vi "SerialPortTest.vi"() -> ()   [LabVIEW 2013]
panel:
  out "error out 2":errorcluster
  out "Buffer":string
  out "error out":errorcluster
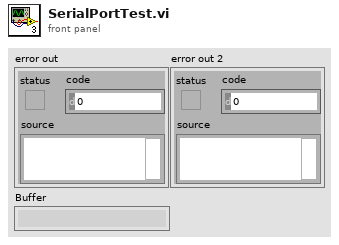
[diagram p1: front panel]
types:
  T1 = typedef "WPI_SerialPortRef.ctl" = cluster{"DevStatus":errorcluster, "Serial Port Name":refnum<visa-resource-name>}
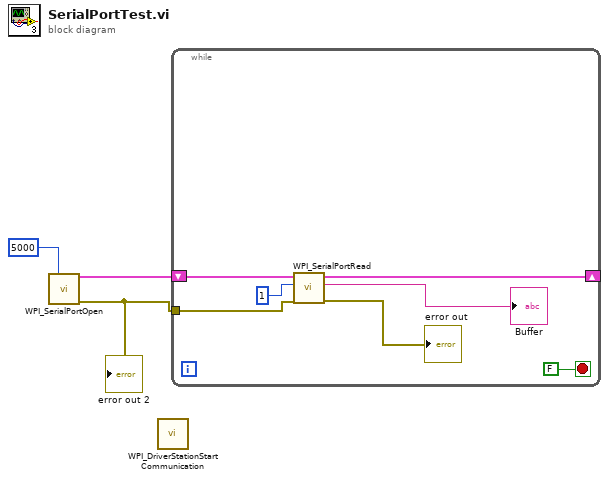
[diagram p0: block diagram]
diagram:
  n1 = call <vilib>:"WPI_SerialPortOpen.vi"("Timeout Value (ms)"=u32 5000) -> ("SerialPortRef"=w3:T1, "error out"=w2:errorcluster)  [unwired: 13 in]
  "error out 2" <- w2
  n2 = call <vilib>:"WPI_DriverStationStart Communication.vi"() -> ()  [unwired: 12 in]
  n3 = while {
    tunnel: w2 -> [w7]
    shift-right: [w4] -> _
    shift-left: w3 -> [w9]
    stop <- FALSE stop-if-true
    n4 = call <vilib>:"WPI_SerialPortRead.vi"("error in (no error)"=w7, "Num Bytes to Read"=u32 1, "SerialPortRef"=w9) -> ("error out"=→"error out":errorcluster, "Buffer"=→"Buffer":string, "SerialPortRef"=w4:T1)  [unwired: 6 in]
  }
